vi "Ivan_method.vi"() -> ()   [LabVIEW 2017]
uses:
  ONNX Class/ONNX Class.lvclass
  <vilib>/Utility/file.llb/Read Delimited Spreadsheet (DBL).vi
panel:
  out "output array":dbl[][][](array[numeric])
  out "Output Buffer":sgl[](array[numeric])
  out "time":u32
  out "Y predicted":dbl
  out "X predicted":dbl
  out "X and Y std":sgl[][](array[numeric])
  out "initialized array 2":sgl[][](array[numeric])
  out "X and Y means":sgl[][](array[numeric])
  out "initialized array":sgl[][](array[numeric])
  out "raw data":dbl[][](array[numeric])
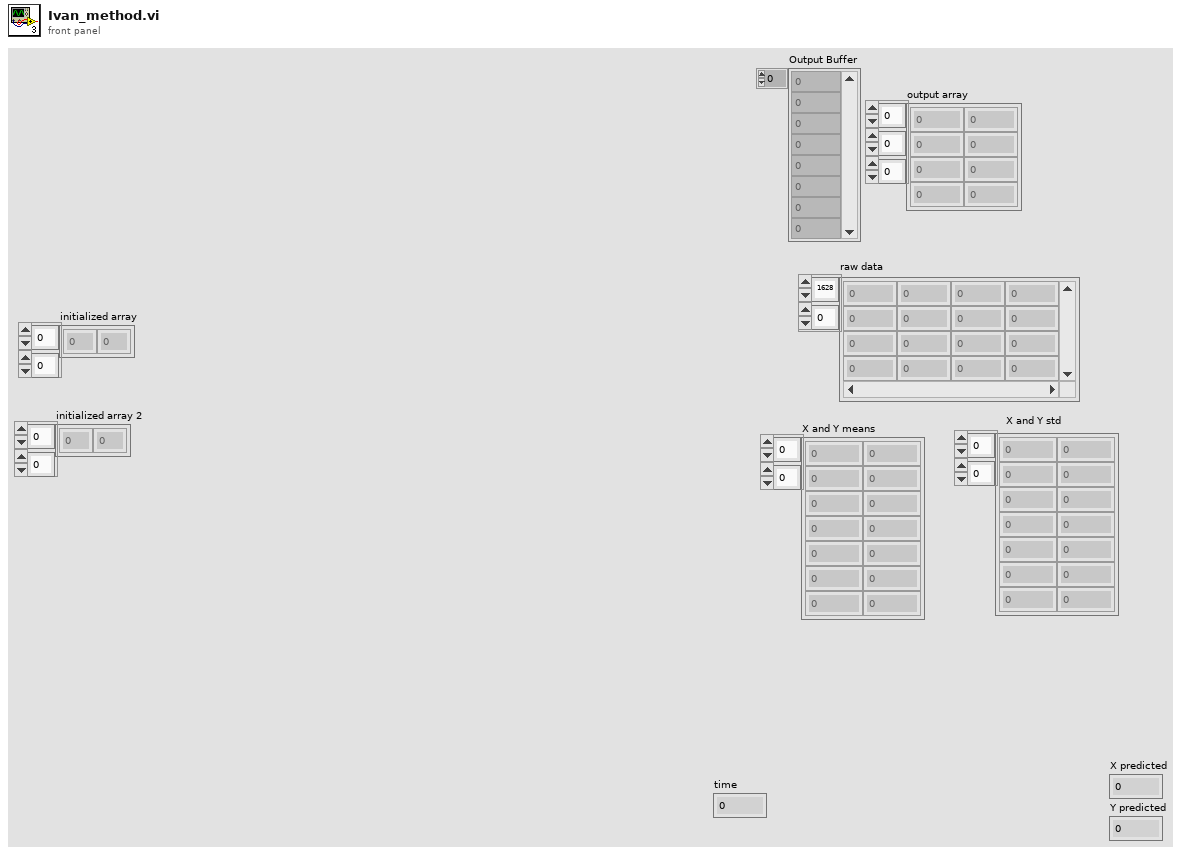
[diagram p1: front panel]
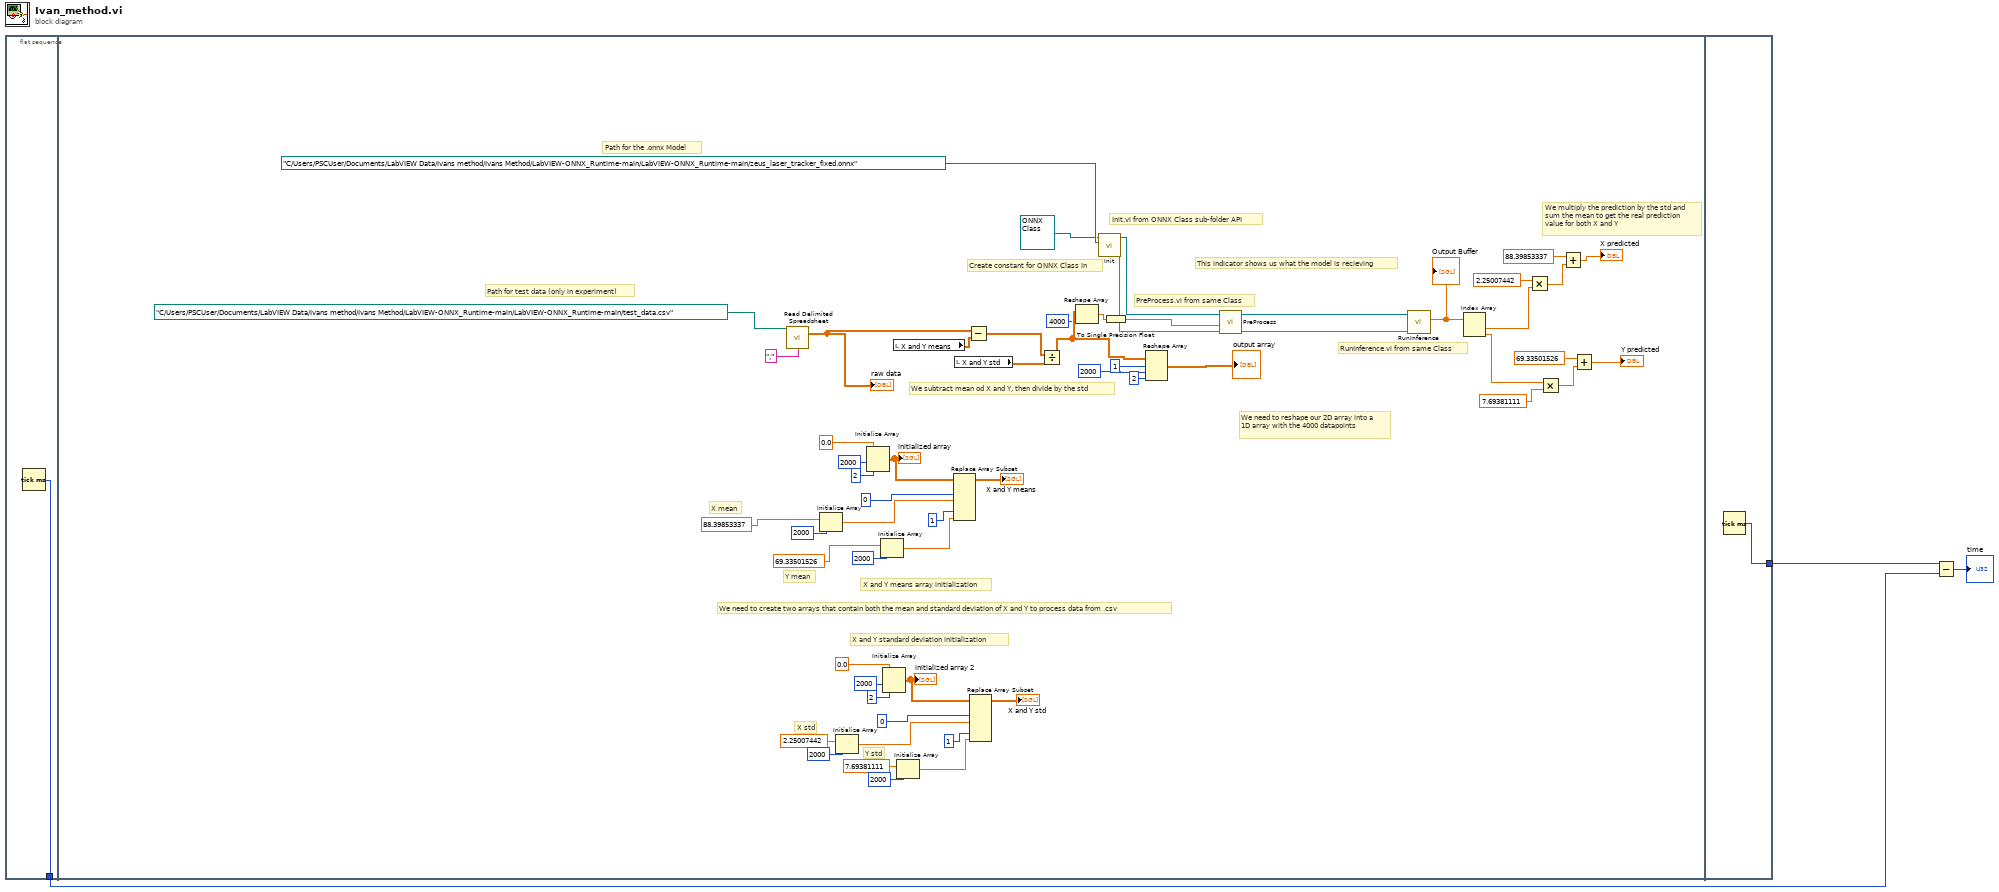
[diagram p0: block diagram]
diagram:
  n1 = flat-sequence {
    tunnel: [w4] -> w2
    tunnel: [w62] -> w3
    frame #0 {
      n2 = Tick Count (ms)() -> (millisecond timer value=w4:u32)
    }
    frame #1 {
      # "We multiply the prediction by the std and sum the mean to get the real prediction value for both X and Y"
      # "This indicator shows us what the model is recieving"
      # "RunInference.vi from same Class"
      # "PreProcess.vi from same Class"
      # "Init.vi from ONNX Class sub-folder API"
      # "Create constant for ONNX Class In"
      # "We need to reshape our 2D array into a 1D array with the 4000 datapoints"
      # "We subtract mean od X and Y, then divide by the std"
      # "Y std"
      # "X std"
      # "Y mean"
      # "X mean"
      # "We need to create two arrays that contain both the mean and standard deviation of X and Y to process data from .csv"
      # "Path for test data (only in experiment)"
      # "Path for the .onnx Model"
      # "X and Y standard deviation initialization"
      # "X and Y means array initialization"
      n3 = call-poly <vilib>:"Read Delimited Spreadsheet.vi"("file path (dialog if empty)"=path "C:/Users/PSCUser/Documents/LabVIEW Data/Ivans method/Ivans Method/LabVIEW-ONNX_Runtime-main/LabVIEW-ONNX_Runtime-main/test_data.csv", "delimiter (\\t)"="," ("delimiter (\\t)")) -> ("all rows"=w48:dbl[][])  [unwired: 8 in, 5 out]
      "raw data" <- w48
      n4 = Initialize Array(88.39853337 ("x"), 2000 ("dimension size")) -> (w51:dbl[])
      n5 = Initialize Array(2.25007442 ("x"), 2000 ("dimension size")) -> (w17:dbl[])
      n6 = Initialize Array(sgl 0.0 ("element"), 2000 ("dimension size"), 2 ("dimension size")) -> (w56:sgl[][])
      "initialized array" <- w56
      n7 = Initialize Array(69.33501526 ("x"), 2000 ("dimension size")) -> (w49:dbl[])
      n8 = Initialize Array(sgl 0.0 ("element"), 2000 ("dimension size"), 2 ("dimension size")) -> (w42:sgl[][])
      "initialized array 2" <- w42
      n9 = local read "X and Y means"() -> (w47:sgl[][])
      n10 = Initialize Array(7.69381111 ("x"), 2000 ("dimension size")) -> (w36:dbl[])
      n11 = Replace Array Subset(array=w56, new element #1=w51, index (col) #1=0 ("disabled index (col)"), new element #2=w49, index (col) #2=1 ("disabled index (col)")) -> (→"X and Y means":sgl[][])  [unwired: 2 in]
      n12 = local read "X and Y std"() -> (w35:sgl[][])
      n13 = Subtract(x=w48, y=w47) -> (x-y=w46:dbl[][])
      n14 = Replace Array Subset(array=w42, new element #1=w17, index (col) #1=0 ("disabled index (col)"), new element #2=w36, index (col) #2=1 ("disabled index (col)")) -> (→"X and Y std":sgl[][])  [unwired: 2 in]
      n15 = Divide(x=w46, y=w35) -> (x/y=w8:dbl[][])
      n16 = Reshape Array(w8, 4000 ("dimension size")) -> (w6:dbl[])
      n17 = call-dynamic "Init.vi"("ONNX Path"=path "C:/Users/PSCUser/Documents/LabVIEW Data/Ivans method/Ivans Method/LabVIEW-ONNX_Runtime-main/LabVIEW-ONNX_Runtime-main/zeus_laser_tracker_fixed.onnx", "ONNX Class in"=refnum<class "ONNX Class.lvclass"> refnum) -> ("error out"=w18:errorcluster, "ONNX Class out"=w19:refnum<class "ONNX Class.lvclass">)  [unwired: 7 in, 1 out]
      n18 = To Single Precision Float(number=w6) -> (single precision float=w5:sgl[])
      n19 = Reshape Array(w8, 1 ("dimension size"), 2000 ("dimension size"), 2 ("dimension size")) -> (→"output array":dbl[][][])
      n20 = call-dynamic "PreProcess.vi"("error in (no error)"=w18, "Array"=w5, "ONNX Class in"=w19) -> ("error out"=w21:errorcluster, "ONNX Class out"=w20:refnum<class "ONNX Class.lvclass">)  [unwired: 6 in, 1 out]
      n21 = call-dynamic "RunInference.vi"("error in (no error)"=w21, "ONNX Class in"=w20) -> ("Output Buffer"=w22:sgl[])  [unwired: 7 in, 2 out]
      "Output Buffer" <- w22
      n22 = Index Array(array=w22) -> (element #1=w26:sgl, element #2=w31:sgl)  [unwired: 2 in]
      n23 = Multiply(x=2.25007442, y=w26) -> (x*y=w25:dbl)
      n24 = Multiply(x=w31, y=7.69381111 ("x")) -> (x*y=w29:dbl)
      n25 = Add(x=88.39853337, y=w25) -> (x+y=→"X predicted":dbl)
      n26 = Add(x=69.33501526, y=w29) -> (x+y=→"Y predicted":dbl)
    }
    frame #2 {
      n27 = Tick Count (ms)() -> (millisecond timer value=w62:u32)
    }
  }
  n28 = Subtract(x=w3, y=w2) -> (x-y=→"time":u32)
